vi "On Once.vi"(1 "Control":bool) -> (0 "On Once":bool)   [LabVIEW 2014]
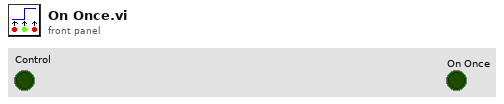
[diagram p1: front panel]
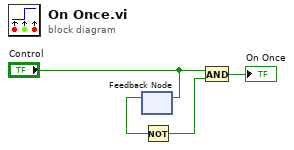
[diagram p0: block diagram]
diagram:
  n1 = feedback-in #1("Control") -> ()
  n2 = feedback #1() -> (w4:bool)  [unwired: 1 in]
  n3 = Not(x=w4) -> (.not. x?=w2:bool)
  n4 = And(x="Control", y=w2) -> (x .and. y?=→"On Once":bool)
